vi "HFRR ADV v034 new software.vi"() -> ()   [LabVIEW 2025] (continued)
          }
        }
      }
    }
    n1885 = case shown="True" "Prog Uno" {
      frame False {
      }
      frame True {
        n1886 = stacked-sequence {
          frame #0 {
            n1887 = Delete(path (use dialog)=path "C:/LAB-IQ-NXT/UNOCOMPILE.bat" ("working directory")) -> ()  [unwired: 4 in, 3 out]
          }
          frame #1 {
            n1888 = local read "Com Port 1"() -> (w2646:refnum<visa-resource-name>)
            n1889 = Concatenate Strings("cmd.exe /c \"mode " ("command line"), w2646, ":1200,n,8,1\"\n" ("command line")) -> (w2651:string)
            n1890 = Concatenate Strings(w2651, "CD\\\nCD WinDucom\navrdude -C avrdude.conf -v -patmega328p -carduino -P" ("command line"), w2646, " -b115200 -D -Uflash:w:UNO_V20.hex:i\n" ("command line"), "\r") -> (w2653:string)
            "STR" <- w2653
            n1891 = call <vilib>:"Write Characters To File.vi"("append to file? (new file:F)"=FALSE, "character string"=w2653, "file path (dialog if empty)"=path "C:/LAB-IQ/UNOCOMPILE.bat" ("working directory")) -> ()  [unwired: 2 in, 1 out]
          }
          frame #2 {
            n1892 = disable-structure shown="Disabled" {
              frame Disabled {
                w2657 = "cmd.exe  /c \"C:\\LAB-IQ-NXT\\UNOCOMPILE.bat\"" ("string")
                n1893 = local write "Prog Uno"(FALSE ("run minimized? (F)")) -> ()
                n1894 = call <vilib>:"System Exec.vi"("expected output size  (4096)"=u32 65535, "run minimized? (F)"=FALSE, "wait until completion? (T)"=TRUE ("run minimized? (F)"), "working directory"=path "C:/LAB-IQ-NXT", "standard input"=w2657, "command line"=w2657) -> ("error out"=w2656:errorcluster, "standard output"=→"String 42":string)  [unwired: 2 in, 2 out]
                "error out 3" <- w2656
                n1895 = flat-sequence {
                  tunnel: w2656 -> [_]
                  frame #0 {
                  }
                }
              }
              frame Enabled {
              }
            }
          }
        }
      }
    }
    n1896 = case shown="\"ISO 12156\"" "TEST STANDARD" {
      frame "ASTM D6079", Default {
        w2626 = 50.0 ("Hz")
        w2627 = 53.0 ("Set Rh")
        w2629 = 1.0 ("Set Strk")
        w2628 = 60.0 ("Set Temp")
        # "astm hide"
        n1897 = local write "NORMAL LOAD"(200.0 ("NORMAL LOAD")) -> ()
        n1898 = local write "Set Strk"(w2629) -> ()
        n1899 = local write "Set Hz"(w2626) -> ()
        n1900 = local write "Set Temp"(w2628) -> ()
        n1901 = local write "Set Rh"(w2627) -> ()
        n1902 = local write "test time"(75.0 ("test time")) -> ()
        n1903 = local write "Set Stroke:"(w2629) -> ()
        n1904 = local write "Set Humidity:"(w2627) -> ()
        n1905 = local write "Set Frequency:"(w2626) -> ()
        n1906 = local write "Set Temperature:"(w2628) -> ()
        "Test Standard" <- "ASTM D6079" ("Test Standard 2")
      }
      frame "ISO 12156" {
        n1907 = local write "Set Strk"(1.0 ("Set Strk")) -> ()
        n1908 = local write "NORMAL LOAD"(200.0 ("NORMAL LOAD")) -> ()
        n1909 = local write "Set Temp"(60.0 ("Set Temp")) -> ()
        n1910 = local write "test time"(75.0 ("test time")) -> ()
        n1911 = local write "Set Hz"(50.0 ("Hz")) -> ()
        n1912 = local write "Set Rh"(53.0 ("Set Rh")) -> ()
      }
      frame "CEC F-096-A-06" {
        n1913 = local write "Set Strk"(1.0 ("Set Strk")) -> ()
        n1914 = local write "NORMAL LOAD"(200.0 ("NORMAL LOAD")) -> ()
        n1915 = local write "Set Temp"(60.0 ("Set Temp")) -> ()
        n1916 = local write "test time"(75.0 ("test time")) -> ()
        n1917 = local write "Set Hz"(50.0 ("Hz")) -> ()
        n1918 = local write "Set Rh"(53.0 ("Set Rh")) -> ()
      }
      frame "Custom" {
      }
    }
    n1919 = Or(x=w2179, y=w2177) -> (x .or. y?=w2178:bool)
    n1920 = case shown="\"About\"" w2176 {
      tunnel: [T28."Acquire" ("Main Tab") T28."Compare Files" ("Main Tab") T28."About" ("Main Tab")] -> w2187
      frame "Acquire", Default {
      }
      frame "Compare Files" {
      }
      frame "About" {
      }
    }
    n1921 = Or(x=w2182, y="OPEN") -> (x .or. y?=w2183:bool)
    n1922 = case shown="True" w2183 {
      tunnel: w2182 -> [_ w2215]
      frame False {
      }
      frame True {
        n1923 = stacked-sequence {
          tunnel: w2215 -> [_ w2282 _ _]
          frame #0 {
            w2231 = "  " ("String 6")
            n1924 = local write "OPEN"(FALSE ("open")) -> ()
            n1925 = local read "string1 2"() -> (w2219:string)
            n1926 = local read "string1 3"() -> (w2218:string)
            n1927 = local read "string1 4"() -> (w2217:string)
            n1928 = property on="OPEN" class="Bool (strict)"("Visible"=FALSE) -> ()  [unwired: 2 in, 2 out]
            n1929 = local write "String 6"(w2231) -> ()
            n1930 = local write "String 7"(w2231) -> ()
            n1931 = local write "String 8"(w2231) -> ()
            n1932 = local write "String 12"(w2231) -> ()
            n1933 = local read "OK Button 16"() -> (w2216:bool)
            n1934 = String To Path(string=w2219) -> (path=w2227:path)
            n1935 = String To Path(string=w2218) -> (path=w2226:path)
            n1936 = String To Path(string=w2217) -> (path=w2225:path)
            n1937 = case shown="True" w2216 {
              tunnel: [w2232 w2233] -> w2220
              frame False {
                n1938 = local read "string1"() -> (w2232:string)
              }
              frame True {
                n1939 = local read "String Indicator 4"() -> (w2233:string)
              }
            }
            n1940 = Open/Create/Replace File "Open File"(file path (use dialog)=w2227) -> (refnum out=w2223:refnum<file>)  [unwired: 5 in, 2 out]
            n1941 = Open/Create/Replace File "Open File"(file path (use dialog)=w2226) -> (refnum out=w2222:refnum<file>)  [unwired: 5 in, 2 out]
            n1942 = Open/Create/Replace File "Open File"(file path (use dialog)=w2225) -> (refnum out=w2221:refnum<file>)  [unwired: 5 in, 2 out]
            n1943 = while {
              tunnel: w2223 -> [w2245]
              i -> [w2241]
              stop <- w2240 continue-if-true
              (unwired) TRUE ("line mode (F)")
              n1944 = Read from Text File "Read File"(file (use dialog)=w2245) -> (text=w2242:string)  [unwired: 3 in, 3 out]
              n1945 = local write "Numeric 11"(w2241) -> ()
              n1946 = String Length(string=w2242) -> (length=w2244:i32)
              n1947 = Greater?(x=w2244, y=1) -> (0:w2240:bool)
            }
            n1948 = while {
              tunnel: w2222 -> [w2251]
              i -> [w2247]
              stop <- w2246 continue-if-true
              (unwired) TRUE ("line mode (F)")
              n1949 = Read from Text File "Read File"(file (use dialog)=w2251) -> (text=w2248:string)  [unwired: 3 in, 3 out]
              n1950 = local write "Numeric 12"(w2247) -> ()
              n1951 = String Length(string=w2248) -> (length=w2250:i32)
              n1952 = Greater?(x=w2250, y=1) -> (0:w2246:bool)
            }
            n1953 = while {
              tunnel: w2221 -> [w2257]
              i -> [w2253]
              stop <- w2252 continue-if-true
              (unwired) TRUE ("line mode (F)")
              n1954 = Read from Text File "Read File"(file (use dialog)=w2257) -> (text=w2254:string)  [unwired: 3 in, 3 out]
              n1955 = local write "Numeric 13"(w2253) -> ()
              n1956 = String Length(string=w2254) -> (length=w2256:i32)
              n1957 = Greater?(x=w2256, y=1) -> (0:w2252:bool)
            }
            n1958 = String To Path(string=w2220) -> (path=w2228:path)
            n1959 = Open/Create/Replace File "Open File"(file path (use dialog)=w2228) -> (refnum out=w2224:refnum<file>)  [unwired: 5 in, 2 out]
            n1960 = while {
              tunnel: w2224 -> [w2239]
              i -> [w2235]
              stop <- w2234 continue-if-true
              (unwired) TRUE ("line mode (F)")
              n1961 = Read from Text File "Read File"(file (use dialog)=w2239) -> (text=w2236:string)  [unwired: 3 in, 3 out]
              n1962 = local write "Numeric 8"(w2235) -> ()
              n1963 = String Length(string=w2236) -> (length=w2238:i32)
              n1964 = Greater?(x=w2238, y=1) -> (0:w2234:bool)
            }
          }
          frame #1 {
            w2409 = FALSE ("ACTUAL   MERGE")
            # "Sample Temp"
            # "ECR"
            # "COF"
            # "Time\nCOF\nFF\nTemp"
            n1965 = case shown="True" w2282 {
              tunnel: [w2429 w2430] -> w2283
              frame False {
                n1966 = local read "string1"() -> (w2429:string)
              }
              frame True {
                n1967 = local read "String Indicator 4"() -> (w2430:string)
              }
            }
            n1968 = local read "string1 3"() -> (w2327:string)
            n1969 = String To Path(string=w2283) -> (path=w2414:path)
            n1970 = String To Path(string=w2327) -> (path=w2425:path)
            n1971 = local read "Numeric 12"() -> (w2411:i32)
            n1972 = local read "Numeric 8"() -> (w2413:i32)
            n1973 = local read "string1 2"() -> (w2328:string)
            n1974 = local read "string1 4"() -> (w2326:string)
            n1975 = Open/Create/Replace File "Open File"(file path (use dialog)=w2414) -> (refnum out=w2428:refnum<file>, error out=w2427:errorcluster)  [unwired: 5 in, 1 out]
            n1976 = Open/Create/Replace File "Open File"(file path (use dialog)=w2425) -> (refnum out=w2421:refnum<file>, error out=w2422:errorcluster)  [unwired: 5 in, 1 out]
            n1977 = for {
              N: w2413 -> [_]
              tunnel: w2428 -> [w2576]
              tunnel: w2427 -> [w2575]
              tunnel: [w2565] -> w2340 mode=indexing
              tunnel: [w2563] -> w2397 mode=indexing
              tunnel: [w2564] -> w2392 mode=indexing
              tunnel: w2409 -> [_]
              tunnel: [w2557] -> w2394 mode=indexing
              tunnel: [w2553] -> w2363 mode=indexing
              tunnel: [w2549] -> w2338 mode=indexing
              tunnel: [w2545] -> w2319 mode=indexing
              tunnel: [w2540] -> w2279 mode=indexing
              (unwired) TRUE ("line mode (F)")
              # "freq"
              # "Stroke"
              # "Time"
              # "CoF"
              # "Humidity"
              # "Temp"
              # "Air Temp"
              # "ECR"
              n1978 = Read from Text File "Read File"(file (use dialog)=w2576, error in=w2575) -> (text=w2541:string)  [unwired: 2 in, 3 out]
              n1979 = local write "String 6"(w2541) -> ()
              n1980 = String Subset(string=w2541, offset (0)=0, length (rest)=14 ("length (rest)")) -> (substring=w2569:string)
              n1981 = String Subset(string=w2541, offset (0)=35, length (rest)=9 ("length (rest)")) -> (substring=w2566:string)
              n1982 = String Subset(string=w2541, offset (0)=15, length (rest)=9 ("length (rest)")) -> (substring=w2572:string)
              n1983 = Fract/Exp String To Number(string=w2569) -> (number=w2565:dbl)  [unwired: 3 in, 1 out]
              n1984 = Fract/Exp String To Number(string=w2566) -> (number=w2564:dbl)  [unwired: 3 in, 1 out]
              n1985 = Fract/Exp String To Number(string=w2572) -> (number=w2563:dbl)  [unwired: 3 in, 1 out]
              n1986 = String Subset(string=w2541, offset (0)=85, length (rest)=9 ("length (rest)")) -> (substring=w2542:string)
              n1987 = String Subset(string=w2541, offset (0)=25, length (rest)=9 ("length (rest)")) -> (substring=w2548:string)
              n1988 = String Subset(string=w2541, offset (0)=55, length (rest)=9 ("length (rest)")) -> (substring=w2550:string)
              n1989 = String Subset(string=w2541, offset (0)=45, length (rest)=9 ("length (rest)")) -> (substring=w2556:string)
              n1990 = String Subset(string=w2541, offset (0)=65, length (rest)=9 ("length (rest)")) -> (substring=w2562:string)
              n1991 = Fract/Exp String To Number(string=w2548) -> (number=w2545:dbl)  [unwired: 3 in, 1 out]
              n1992 = Fract/Exp String To Number(string=w2542) -> (number=w2540:dbl)  [unwired: 3 in, 1 out]
              n1993 = Fract/Exp String To Number(string=w2550) -> (number=w2549:dbl)  [unwired: 3 in, 1 out]
              n1994 = Fract/Exp String To Number(string=w2556) -> (number=w2553:dbl)  [unwired: 3 in, 1 out]
              n1995 = Fract/Exp String To Number(string=w2562) -> (number=w2559:dbl)  [unwired: 3 in, 1 out]
              n1996 = Add(x=w2559, y=0.0) -> (x+y=w2557:dbl)
            }
            n1997 = for {
              N: w2411 -> [_]
              tunnel: w2422 -> [w2502]
              tunnel: w2421 -> [w2501]
              tunnel: [w2491] -> w2380 mode=indexing
              tunnel: [w2489] -> w2378 mode=indexing
              tunnel: [w2490] -> w2374 mode=indexing
              tunnel: w2409 -> [_]
              tunnel: [w2483] -> w2376 mode=indexing
              tunnel: [w2479] -> w2358 mode=indexing
              tunnel: [w2475] -> w2334 mode=indexing
              tunnel: [w2472] -> w2315 mode=indexing
              tunnel: [w2468] -> w2274 mode=indexing
              (unwired) 9 ("length (rest)")
              (unwired) 9 ("length (rest)")
              (unwired) TRUE ("line mode (F)")
              n1998 = Read from Text File "Read File"(file (use dialog)=w2501, error in=w2502) -> (text=w2469:string)  [unwired: 2 in, 3 out]
              n1999 = local write "String 8"(w2469) -> ()
              n2000 = String Subset(string=w2469, offset (0)=85) -> (substring=w2471:string)  [unwired: 1 in]
              n2001 = String Subset(string=w2469, offset (0)=35, length (rest)=9 ("length (rest)")) -> (substring=w2492:string)
              n2002 = String Subset(string=w2469, offset (0)=55, length (rest)=9 ("length (rest)")) -> (substring=w2477:string)
              n2003 = String Subset(string=w2469, offset (0)=25) -> (substring=w2473:string)  [unwired: 1 in]
              n2004 = String Subset(string=w2469, offset (0)=15, length (rest)=9 ("length (rest)")) -> (substring=w2498:string)
              n2005 = String Subset(string=w2469, offset (0)=0, length (rest)=14 ("length (rest)")) -> (substring=w2495:string)
              n2006 = String Subset(string=w2469, offset (0)=45, length (rest)=9 ("length (rest)")) -> (substring=w2482:string)
              n2007 = String Subset(string=w2469, offset (0)=65, length (rest)=9 ("length (rest)")) -> (substring=w2488:string)
              n2008 = Fract/Exp String To Number(string=w2471) -> (number=w2468:dbl)  [unwired: 3 in, 1 out]
              n2009 = Fract/Exp String To Number(string=w2492) -> (number=w2490:dbl)  [unwired: 3 in, 1 out]
              n2010 = Fract/Exp String To Number(string=w2477) -> (number=w2475:dbl)  [unwired: 3 in, 1 out]
              n2011 = Fract/Exp String To Number(string=w2473) -> (number=w2472:dbl)  [unwired: 3 in, 1 out]
              n2012 = Fract/Exp String To Number(string=w2498) -> (number=w2489:dbl)  [unwired: 3 in, 1 out]
              n2013 = Fract/Exp String To Number(string=w2495) -> (number=w2491:dbl)  [unwired: 3 in, 1 out]
              n2014 = Fract/Exp String To Number(string=w2482) -> (number=w2479:dbl)  [unwired: 3 in, 1 out]
              n2015 = Fract/Exp String To Number(string=w2488) -> (number=w2485:dbl)  [unwired: 3 in, 1 out]
              n2016 = Add(x=w2485, y=0.0) -> (x+y=w2483:dbl)
            }
            n2017 = String To Path(string=w2328) -> (path=w2426:path)
            n2018 = String To Path(string=w2326) -> (path=w2420:path)
            n2019 = local read "Numeric 11"() -> (w2410:i32)
            n2020 = local read "Numeric 13"() -> (w2412:i32)
            n2021 = Open/Create/Replace File "Open File"(file path (use dialog)=w2426) -> (refnum out=w2424:refnum<file>, error out=w2423:errorcluster)  [unwired: 5 in, 1 out]
            n2022 = Open/Create/Replace File "Open File"(file path (use dialog)=w2420) -> (refnum out=w2419:refnum<file>, error out=w2418:errorcluster)  [unwired: 5 in, 1 out]
            n2023 = for {
              N: w2410 -> [_]
              tunnel: w2424 -> [w2539]
              tunnel: w2423 -> [w2538]
              tunnel: [w2528] -> w2390 mode=indexing
              tunnel: [w2526] -> w2388 mode=indexing
              tunnel: [w2527] -> w2383 mode=indexing
              tunnel: w2409 -> [_]
              tunnel: [w2520] -> w2385 mode=indexing
              tunnel: [w2516] -> w2361 mode=indexing
              tunnel: [w2512] -> w2336 mode=indexing
              tunnel: [w2508] -> w2317 mode=indexing
              tunnel: [w2503] -> w2275 mode=indexing
              (unwired) TRUE ("line mode (F)")
              n2024 = Read from Text File "Read File"(file (use dialog)=w2539, error in=w2538) -> (text=w2504:string)  [unwired: 2 in, 3 out]
              n2025 = local write "String 7"(w2504) -> ()
              n2026 = String Subset(string=w2504, offset (0)=85, length (rest)=9 ("length (rest)")) -> (substring=w2507:string)
              n2027 = String Subset(string=w2504, offset (0)=35, length (rest)=9 ("length (rest)")) -> (substring=w2529:string)
              n2028 = String Subset(string=w2504, offset (0)=55, length (rest)=9 ("length (rest)")) -> (substring=w2515:string)
              n2029 = String Subset(string=w2504, offset (0)=25, length (rest)=9 ("length (rest)")) -> (substring=w2509:string)
              n2030 = String Subset(string=w2504, offset (0)=45, length (rest)=9 ("length (rest)")) -> (substring=w2517:string)
              n2031 = String Subset(string=w2504, offset (0)=0, length (rest)=14 ("length (rest)")) -> (substring=w2532:string)
              n2032 = String Subset(string=w2504, offset (0)=15, length (rest)=9 ("length (rest)")) -> (substring=w2535:string)
              n2033 = String Subset(string=w2504, offset (0)=65, length (rest)=9 ("length (rest)")) -> (substring=w2521:string)
              n2034 = Fract/Exp String To Number(string=w2507) -> (number=w2503:dbl)  [unwired: 3 in, 1 out]
              n2035 = Fract/Exp String To Number(string=w2529) -> (number=w2527:dbl)  [unwired: 3 in, 1 out]
              n2036 = Fract/Exp String To Number(string=w2515) -> (number=w2512:dbl)  [unwired: 3 in, 1 out]
              n2037 = Fract/Exp String To Number(string=w2509) -> (number=w2508:dbl)  [unwired: 3 in, 1 out]
              n2038 = Fract/Exp String To Number(string=w2517) -> (number=w2516:dbl)  [unwired: 3 in, 1 out]
              n2039 = Fract/Exp String To Number(string=w2532) -> (number=w2528:dbl)  [unwired: 3 in, 1 out]
              n2040 = Fract/Exp String To Number(string=w2535) -> (number=w2526:dbl)  [unwired: 3 in, 1 out]
              n2041 = Fract/Exp String To Number(string=w2521) -> (number=w2524:dbl)  [unwired: 3 in, 1 out]
              n2042 = Add(x=w2524, y=0.0) -> (x+y=w2520:dbl)
            }
            n2043 = for {
              N: w2412 -> [_]
              tunnel: w2419 -> [w2467]
              tunnel: w2418 -> [w2466]
              tunnel: [w2456] -> w2372 mode=indexing
              tunnel: [w2455] -> w2365 mode=indexing
              tunnel: w2409 -> [_]
              tunnel: [w2444] -> w2370 mode=indexing
              tunnel: [w2449] -> w2367 mode=indexing
              tunnel: [w2445] -> w2357 mode=indexing
              tunnel: [w2440] -> w2332 mode=indexing
              tunnel: [w2436] -> w2313 mode=indexing
              tunnel: [w2431] -> w2273 mode=indexing
              (unwired) 1.0 ("x")
              (unwired) TRUE ("line mode (F)")
              n2044 = Read from Text File "Read File"(file (use dialog)=w2467, error in=w2466) -> (text=w2432:string)  [unwired: 2 in, 3 out]
              n2045 = local write "String 12"(w2432) -> ()
              n2046 = String Subset(string=w2432, offset (0)=85, length (rest)=9 ("length (rest)")) -> (substring=w2434:string)
              n2047 = String Subset(string=w2432, offset (0)=35, length (rest)=9 ("length (rest)")) -> (substring=w2457:string)
              n2048 = String Subset(string=w2432, offset (0)=55, length (rest)=9 ("length (rest)")) -> (substring=w2442:string)
              n2049 = String Subset(string=w2432, offset (0)=25, length (rest)=9 ("length (rest)")) -> (substring=w2438:string)
              n2050 = String Subset(string=w2432, offset (0)=45, length (rest)=9 ("length (rest)")) -> (substring=w2447:string)
              n2051 = String Subset(string=w2432, offset (0)=15, length (rest)=9 ("length (rest)")) -> (substring=w2463:string)
              n2052 = String Subset(string=w2432, offset (0)=0, length (rest)=14 ("length (rest)")) -> (substring=w2460:string)
              n2053 = String Subset(string=w2432, offset (0)=65, length (rest)=9 ("length (rest)")) -> (substring=w2450:string)
              n2054 = Fract/Exp String To Number(string=w2434) -> (number=w2431:dbl)  [unwired: 3 in, 1 out]
              n2055 = Fract/Exp String To Number(string=w2457) -> (number=w2455:dbl)  [unwired: 3 in, 1 out]
              n2056 = Fract/Exp String To Number(string=w2442) -> (number=w2440:dbl)  [unwired: 3 in, 1 out]
              n2057 = Fract/Exp String To Number(string=w2438) -> (number=w2436:dbl)  [unwired: 3 in, 1 out]
              n2058 = Fract/Exp String To Number(string=w2447) -> (number=w2445:dbl)  [unwired: 3 in, 1 out]
              n2059 = Fract/Exp String To Number(string=w2463) -> (number=w2444:dbl)  [unwired: 3 in, 1 out]
              n2060 = Fract/Exp String To Number(string=w2460) -> (number=w2456:dbl)  [unwired: 3 in, 1 out]
              n2061 = Fract/Exp String To Number(string=w2450) -> (number=w2453:dbl)  [unwired: 3 in, 1 out]
              n2062 = Add(x=w2453, y=0.0) -> (x+y=w2449:dbl)
            }
            n2063 = Delete From Array(array=w2315, index=0) -> (array with subset deleted=w2288:dbl[])  [unwired: 1 in, 1 out]
            n2064 = Delete From Array(array=w2378, index=0) -> (array with subset deleted=w2351:dbl[])  [unwired: 1 in, 1 out]
            n2065 = Delete From Array(array=w2358, index=0) -> (array with subset deleted=w2346:dbl[])  [unwired: 1 in, 1 out]
            n2066 = Delete From Array(array=w2376, index=0) -> (array with subset deleted=w2377:dbl[])  [unwired: 1 in, 1 out]
            n2067 = call-poly <vilib>:"Mean.vi"("X"=w2288) -> ("mean"=→"КОФ2 4":dbl)  [unwired: 1 out]
            n2068 = call-poly <vilib>:"Mean.vi"("X"=w2351) -> ("mean"=→"КОФ3":dbl)  [unwired: 1 out]
            n2069 = call-poly <vilib>:"Mean.vi"("X"=w2346) -> ("mean"=→"CP3":dbl)  [unwired: 1 out]
            n2070 = Delete From Array(array=w2340, index=0) -> (array with subset deleted=w2267:dbl[])  [unwired: 1 in, 1 out]
            n2071 = Delete From Array(array=w2279, index=0) -> (array with subset deleted=w2266:dbl[])  [unwired: 1 in, 1 out]
            n2072 = Delete From Array(array=w2319, index=0) -> (array with subset deleted=w2290:dbl[])  [unwired: 1 in, 1 out]
            n2073 = Delete From Array(array=w2397, index=0) -> (array with subset deleted=w2352:dbl[])  [unwired: 1 in, 1 out]
            n2074 = Delete From Array(array=w2363, index=0) -> (array with subset deleted=w2348:dbl[])  [unwired: 1 in, 1 out]
            "array w/ subset deleted" <- w2348
            n2075 = Delete From Array(array=w2394, index=0) -> (array with subset deleted=w2395:dbl[])  [unwired: 1 in, 1 out]
            n2076 = call-poly <vilib>:"Mean.vi"("X"=w2290) -> ("mean"=→"КОФ2 2":dbl)  [unwired: 1 out]
            n2077 = call-poly <vilib>:"Mean.vi"("X"=w2352) -> ("mean"=→"КОФ1":dbl)  [unwired: 1 out]
            n2078 = Bundle "Bundle"(w2267, w2266) -> (w2272:cluster{dbl[], dbl[]})  [unwired: 1 in]
            n2079 = Bundle "Bundle"(w2267, w2395) -> (w2259:cluster{dbl[], dbl[]})  [unwired: 1 in]
            n2080 = Delete From Array(array=w2274, index=0) -> (array with subset deleted=w2262:dbl[])  [unwired: 1 in, 1 out]
            n2081 = Delete From Array(array=w2275, index=0) -> (array with subset deleted=w2264:dbl[])  [unwired: 1 in, 1 out]
            n2082 = Delete From Array(array=w2385, index=0) -> (array with subset deleted=w2386:dbl[])  [unwired: 1 in, 1 out]
            n2083 = Delete From Array(array=w2273, index=0) -> (array with subset deleted=w2260:dbl[])  [unwired: 1 in, 1 out]
            n2084 = Delete From Array(array=w2367, index=0) -> (array with subset deleted=w2368:dbl[])  [unwired: 1 in, 1 out]
            n2085 = Delete From Array(array=w2392, index=0) -> (array with subset deleted=w2298:dbl[])  [unwired: 1 in, 1 out]
            n2086 = Delete From Array(array=w2338, index=0) -> (array with subset deleted=w2294:dbl[])  [unwired: 1 in, 1 out]
            n2087 = Delete From Array(array=w2374, index=0) -> (array with subset deleted=w2296:dbl[])  [unwired: 1 in, 1 out]
            n2088 = Delete From Array(array=w2334, index=0) -> (array with subset deleted=w2292:dbl[])  [unwired: 1 in, 1 out]
            n2089 = Delete From Array(array=w2383, index=0) -> (array with subset deleted=w2297:dbl[])  [unwired: 1 in, 1 out]
            n2090 = Delete From Array(array=w2336, index=0) -> (array with subset deleted=w2293:dbl[])  [unwired: 1 in, 1 out]
            n2091 = Delete From Array(array=w2317, index=0) -> (array with subset deleted=w2289:dbl[])  [unwired: 1 in, 1 out]
            n2092 = Delete From Array(array=w2361, index=0) -> (array with subset deleted=w2347:dbl[])  [unwired: 1 in, 1 out]
            n2093 = Delete From Array(array=w2388, index=0) -> (array with subset deleted=w2349:dbl[])  [unwired: 1 in, 1 out]
            n2094 = Delete From Array(array=w2365, index=0) -> (array with subset deleted=w2295:dbl[])  [unwired: 1 in, 1 out]
            n2095 = Delete From Array(array=w2332, index=0) -> (array with subset deleted=w2291:dbl[])  [unwired: 1 in, 1 out]
            n2096 = Delete From Array(array=w2313, index=0) -> (array with subset deleted=w2287:dbl[])  [unwired: 1 in, 1 out]
            n2097 = Delete From Array(array=w2357, index=0) -> (array with subset deleted=w2345:dbl[])  [unwired: 1 in, 1 out]
            n2098 = Delete From Array(array=w2370, index=0) -> (array with subset deleted=w2350:dbl[])  [unwired: 1 in, 1 out]
            n2099 = Delete From Array(array=w2380, index=0) -> (array with subset deleted=w2263:dbl[])  [unwired: 1 in, 1 out]
            n2100 = Delete From Array(array=w2390, index=0) -> (array with subset deleted=w2265:dbl[])  [unwired: 1 in, 1 out]
            n2101 = Delete From Array(array=w2372, index=0) -> (array with subset deleted=w2261:dbl[])  [unwired: 1 in, 1 out]
            n2102 = Bundle "Bundle"(w2267, w2298) -> (w2285:cluster{dbl[], dbl[]})  [unwired: 1 in]
            n2103 = Bundle "Bundle"(w2267, w2352) -> (w2286:cluster{dbl[], dbl[]})  [unwired: 1 in]
            n2104 = Bundle "Bundle"(w2298, w2294) -> (w2300:cluster{dbl[], dbl[]})  [unwired: 1 in]
            n2105 = Bundle "Bundle"(w2263, w2262) -> (w2270:cluster{dbl[], dbl[]})  [unwired: 1 in]
            n2106 = Bundle "Bundle"(w2296, w2292) -> (w2302:cluster{dbl[], dbl[]})  [unwired: 1 in]
            n2107 = Bundle "Bundle"(w2263, w2296) -> (w2406:cluster{dbl[], dbl[]})  [unwired: 1 in]
            n2108 = Bundle "Bundle"(w2263, w2292) -> (w2330:cluster{dbl[], dbl[]})  [unwired: 1 in]
            n2109 = Bundle "Bundle"(w2263, w2351) -> (w2416:cluster{dbl[], dbl[]})  [unwired: 1 in]
            n2110 = Bundle "Bundle"(w2263, w2346) -> (w2354:cluster{dbl[], dbl[]})  [unwired: 1 in]
            n2111 = Bundle "Bundle"(w2263, w2377) -> (w2401:cluster{dbl[], dbl[]})  [unwired: 1 in]
            n2112 = Bundle "Bundle"(w2297, w2293) -> (w2301:cluster{dbl[], dbl[]})  [unwired: 1 in]
            n2113 = Bundle "Bundle"(w2265, w2264) -> (w2271:cluster{dbl[], dbl[]})  [unwired: 1 in]
            n2114 = Bundle "Bundle"(w2265, w2297) -> (w2408:cluster{dbl[], dbl[]})  [unwired: 1 in]
            n2115 = Bundle "Bundle"(w2265, w2293) -> (w2331:cluster{dbl[], dbl[]})  [unwired: 1 in]
            n2116 = Bundle "Bundle"(w2265, w2347) -> (w2355:cluster{dbl[], dbl[]})  [unwired: 1 in]
            n2117 = Bundle "Bundle"(w2265, w2349) -> (w2417:cluster{dbl[], dbl[]})  [unwired: 1 in]
            n2118 = Bundle "Bundle"(w2265, w2386) -> (w2399:cluster{dbl[], dbl[]})  [unwired: 1 in]
            n2119 = Bundle "Bundle"(w2295, w2291) -> (w2303:cluster{dbl[], dbl[]})  [unwired: 1 in]
            n2120 = Bundle "Bundle"(w2261, w2260) -> (w2269:cluster{dbl[], dbl[]})  [unwired: 1 in]
            n2121 = Bundle "Bundle"(w2261, w2295) -> (w2407:cluster{dbl[], dbl[]})  [unwired: 1 in]
            n2122 = Bundle "Bundle"(w2261, w2291) -> (w2329:cluster{dbl[], dbl[]})  [unwired: 1 in]
            n2123 = Bundle "Bundle"(w2261, w2345) -> (w2353:cluster{dbl[], dbl[]})  [unwired: 1 in]
            n2124 = Bundle "Bundle"(w2261, w2350) -> (w2415:cluster{dbl[], dbl[]})  [unwired: 1 in]
            n2125 = Bundle "Bundle"(w2261, w2368) -> (w2400:cluster{dbl[], dbl[]})  [unwired: 1 in]
            n2126 = call-poly <vilib>:"Mean.vi"("X"=w2348) -> ("mean"=→"CP1":dbl)  [unwired: 1 out]
            n2127 = call-poly <vilib>:"Mean.vi"("X"=w2289) -> ("mean"=→"КОФ2 3":dbl)  [unwired: 1 out]
            n2128 = call-poly <vilib>:"Mean.vi"("X"=w2347) -> ("mean"=→"CP2":dbl)  [unwired: 1 out]
            n2129 = call-poly <vilib>:"Mean.vi"("X"=w2349) -> ("mean"=→"КОФ2":dbl)  [unwired: 1 out]
            n2130 = call-poly <vilib>:"Mean.vi"("X"=w2287) -> ("mean"=→"КОФ2 5":dbl)  [unwired: 1 out]
            n2131 = call-poly <vilib>:"Mean.vi"("X"=w2345) -> ("mean"=→"CP4":dbl)  [unwired: 1 out]
            n2132 = call-poly <vilib>:"Mean.vi"("X"=w2350) -> ("mean"=→"КОФ4":dbl)  [unwired: 1 out]
            n2133 = Bundle "Bundle"(w2267, w2294) -> (w2258:cluster{dbl[], dbl[]})  [unwired: 1 in]
            n2134 = Bundle "Bundle"(w2267, w2348) -> (w2281:cluster{dbl[], dbl[]})  [unwired: 1 in]
            n2135 = Build Array "Build Array"(w2258, w2281) -> (w2284:cluster{dbl[], dbl[]}[])
            "XY Graph 17" <- w2284
            n2136 = Build Array "Build Array"(w2272, w2271, w2270, w2269) -> (→"Frequency ( Hz )":cluster{dbl[], dbl[]}[])
            n2137 = Build Array "Build Array"(w2300, w2301, w2302, w2303) -> (→"Air Temp ( °C ) vs Humidity ( % RH )":cluster{dbl[], dbl[]}[])
            n2138 = Build Array "Build Array"(w2285, w2408, w2406, w2407) -> (→"Air Temperature  ( °C )":cluster{dbl[], dbl[]}[])
            n2139 = Build Array "Build Array"(w2258, w2331, w2330, w2329) -> (→"Humidity ( %RH )":cluster{dbl[], dbl[]}[])
            n2140 = Build Array "Build Array"(w2286, w2417, w2416, w2415) -> (→"Coefficient Of Friction":cluster{dbl[], dbl[]}[])
            n2141 = Build Array "Build Array"(w2281, w2355, w2354, w2353) -> (→"Sample Temperature ( °C )":cluster{dbl[], dbl[]}[])
            n2142 = Build Array "Build Array"(w2259, w2399, w2401, w2400) -> (→"XY Graph 13":cluster{dbl[], dbl[]}[])
            n2143 = Bundle "Bundle"(w2267, w2290) -> (w2312:cluster{dbl[], dbl[]})  [unwired: 1 in]
            n2144 = Bundle "Bundle"(w2263, w2288) -> (w2310:cluster{dbl[], dbl[]})  [unwired: 1 in]
            n2145 = Bundle "Bundle"(w2265, w2289) -> (w2311:cluster{dbl[], dbl[]})  [unwired: 1 in]
            n2146 = Bundle "Bundle"(w2261, w2287) -> (w2309:cluster{dbl[], dbl[]})  [unwired: 1 in]
            n2147 = Build Array "Build Array"(w2312, w2311, w2310, w2309) -> (→"Stroke ( mm )":cluster{dbl[], dbl[]}[])
            n2148 = local write "XY Graph 16"(w2284) -> ()
          }
          frame #2 {
          }
          frame #3 {
            n2149 = local write "Numeric 8"(0 ("Numeric 8")) -> ()
            n2150 = local write "Numeric 11"(0 ("Numeric 11")) -> ()
            n2151 = local write "Numeric 12"(0 ("Numeric 12")) -> ()
            n2152 = local write "Numeric 13"(0 ("Numeric 13")) -> ()
            n2153 = property on="OPEN" class="Bool (strict)"("Visible"=TRUE) -> ()  [unwired: 2 in, 2 out]
            n2154 = local read "String Control 2"() -> (w2584:string)
            n2155 = local read "String Control 4"() -> (w2583:string)
            n2156 = local read "String Control 6"() -> (w2582:string)
            n2157 = local read "String Control 8"() -> (w2581:string)
            n2158 = Match Pattern(string=w2584, regular expression="Samples / cycle :- ") -> (after substring=w2598:string)  [unwired: 1 in, 3 out]
            n2159 = Match Pattern(string=w2584, regular expression="Frequency :- ") -> (after substring=w2617:string)  [unwired: 1 in, 3 out]
            n2160 = Match Pattern(string=w2583, regular expression="Samples / cycle :- ") -> (after substring=w2594:string)  [unwired: 1 in, 3 out]
            n2161 = Match Pattern(string=w2583, regular expression="Frequency :- ") -> (after substring=w2612:string)  [unwired: 1 in, 3 out]
            n2162 = Match Pattern(string=w2582, regular expression="Samples / cycle :- ") -> (after substring=w2590:string)  [unwired: 1 in, 3 out]
            n2163 = Match Pattern(string=w2582, regular expression="Frequency :- ") -> (after substring=w2607:string)  [unwired: 1 in, 3 out]
            n2164 = Match Pattern(string=w2581, regular expression="Samples / cycle :- ") -> (after substring=w2586:string)  [unwired: 1 in, 3 out]
            n2165 = Match Pattern(string=w2581, regular expression="Frequency :- ") -> (after substring=w2602:string)  [unwired: 1 in, 3 out]
            n2166 = String Subset(string=w2598, length (rest)=6 ("length (rest)")) -> (substring=w2600:string)  [unwired: 1 in]
            n2167 = String Subset(string=w2617, length (rest)=9 ("length (rest)")) -> (substring=w2619:string)  [unwired: 1 in]
            n2168 = String Subset(string=w2594, length (rest)=6 ("length (rest)")) -> (substring=w2596:string)  [unwired: 1 in]
            n2169 = String Subset(string=w2612, length (rest)=9 ("length (rest)")) -> (substring=w2614:string)  [unwired: 1 in]
            n2170 = String Subset(string=w2590, length (rest)=6 ("length (rest)")) -> (substring=w2592:string)  [unwired: 1 in]
            n2171 = String Subset(string=w2607, length (rest)=9 ("length (rest)")) -> (substring=w2609:string)  [unwired: 1 in]
            n2172 = String Subset(string=w2586, length (rest)=6 ("length (rest)")) -> (substring=w2588:string)  [unwired: 1 in]
            n2173 = String Subset(string=w2602, length (rest)=9 ("length (rest)")) -> (substring=w2604:string)  [unwired: 1 in]
            n2174 = Fract/Exp String To Number(string=w2600) -> (number=w2580:dbl)  [unwired: 3 in, 1 out]
            n2175 = Fract/Exp String To Number(string=w2619) -> (number=w2620:dbl)  [unwired: 3 in, 1 out]
            n2176 = Fract/Exp String To Number(string=w2596) -> (number=w2579:dbl)  [unwired: 3 in, 1 out]
            n2177 = Fract/Exp String To Number(string=w2614) -> (number=w2615:dbl)  [unwired: 3 in, 1 out]
            n2178 = Fract/Exp String To Number(string=w2592) -> (number=w2578:dbl)  [unwired: 3 in, 1 out]
            n2179 = Fract/Exp String To Number(string=w2609) -> (number=w2610:dbl)  [unwired: 3 in, 1 out]
            n2180 = Fract/Exp String To Number(string=w2588) -> (number=w2577:dbl)  [unwired: 3 in, 1 out]
            n2181 = Fract/Exp String To Number(string=w2604) -> (number=w2605:dbl)  [unwired: 3 in, 1 out]
            n2182 = local write "sample1"(w2580) -> ()
            n2183 = local write "freq1"(w2620) -> ()
            n2184 = local write "sample2"(w2579) -> ()
            n2185 = local write "freq2"(w2615) -> ()
            n2186 = local write "sample3"(w2578) -> ()
            n2187 = local write "freq3"(w2610) -> ()
            n2188 = local write "sample4"(w2577) -> ()
            n2189 = local write "freq 4"(w2605) -> ()
          }
        }
      }
    }
    n2190 = case shown="True" w2178 {
      selector: w2178 -> [_ w2197]
      frame False {
      }
      frame True {
        n2191 = Not(x=w2197) -> (.not. x?=w2193:bool)
        n2192 = local write "service 3"(w2193) -> ()
        n2193 = local write "OPEN 6"(w2193) -> ()
        n2194 = call <vilib>:"System Exec.vi"("wait until completion? (T)"=TRUE, "command line"="C:\\LAB-IQ\\Scar View.exe") -> ("error out"=→"error out 5":errorcluster)  [unwired: 6 in, 3 out]
      }
    }
    n2195 = case shown="\"Acquire\", Default" w2187 {
      frame "Acquire", Default {
        # "Elapsed time\ncof\nstroke\nAir temp\nTemp\nHumidity"
        n2196 = disable-structure shown="Disabled" {
          frame Disabled {
            n2197 = local read "Flag"() -> (w2896:dbl)
            n2198 = local read "RUN"() -> (w2893:bool)
            n2199 = Not(x=w2893) -> (.not. x?=w2892:bool)
            n2200 = Equal?(x=w2896, y=10.0) -> (x = y?=w2894:bool)
            n2201 = And(x=w2894, y=w2892) -> (x .and. y?=w2891:bool)
            n2202 = case shown="True" w2891 {
              frame False {
              }
              frame True {
                w2897 = FALSE ("Heater Button")
                n2203 = local write "Humidity"(w2897) -> ()
                n2204 = local write "Heater Button"(w2897) -> ()
              }
            }
          }
          frame Enabled {
          }
        }
        n2205 = disable-structure shown="Disabled" {
          frame Disabled {
            n2206 = case shown="True" {
              selector: _ -> [_ _]
              frame False {
              }
              frame True {
                w2950 = TRUE ("Heater")
                n2207 = local write "Humidity"(w2950) -> ()
                n2208 = local write "Heater Button"(w2950) -> ()
                n2209 = local read "TEST STANDARD"() -> (w2953:T3)
                n2210 = local read "TEST STANDARD"() -> (w2948:T3)
                n2211 = Equal?(x=w2953, y=enum16{"ASTM D6079", "ISO 12156", "Custom"}."ISO 12156" ("Test Standard")) -> (x = y?=w2951:bool)
                n2212 = Equal?(x=w2948, y=enum16{"ASTM D6079", "ISO 12156", "Custom"}."ASTM D6079" ("Test Standard")) -> (x = y?=w2947:bool)
                n2213 = case shown="True" w2951 {
                  frame False {
                  }
                  frame True {
                    n2214 = local write "airtempflg"(FALSE ("airtempflg")) -> ()
                    n2215 = local write item#-1(TRUE ("Heater")) -> ()
                  }
                }
                n2216 = case shown="True" w2947 {
                  frame False {
                  }
                  frame True {
                    n2217 = local write "airtempflg"(TRUE ("airtempflg")) -> ()
                    n2218 = local write item#-1(FALSE ("Heater")) -> ()
                  }
                }
              }
            }
          }
          frame Enabled {
          }
        }
        n2219 = stacked-sequence {
          frame #0 {
            n2220 = case shown="True" "RST FF" {
              frame False {
              }
              frame True {
                w2967 = 0.0 ("X Scale.Range:Maximum")
                n2221 = property on="Frictional Force ( N )" class="WFChart (strict)"("XScale.Maximum"=600.0 ("X Scale.Range:Maximum"), "XScale.Minimum"=w2967, "YScale.Maximum"=10.0 ("Y Scale.Range:Maximum"), "YScale.Minimum"=w2967) -> ()  [unwired: 2 in, 2 out]
              }
            }
          }
          frame #1 {
            n2222 = case shown="True" "RST TEMP" {
              frame False {
              }
              frame True {
                n2223 = property on="Temperature ( Deg C )" class="WFChart (strict)"("XScale.Minimum"=0.0 ("X Scale.Range:Minimum"), "XScale.Maximum"=600.0 ("X Scale.Range:Maximum"), "YScale.Minimum"=0.0 ("Y Scale.Range:Minimum"), "YScale.Maximum"=100.0 ("Y Scale.Range:Maximum")) -> ()  [unwired: 2 in, 2 out]
              }
            }
          }
          frame #2 {
            n2224 = case shown="True" "RSTCOF" {
              frame False {
              }
              frame True {
                n2225 = property on="Coefficient of Friction" class="WFChart (strict)"("XScale.Minimum"=0.0 ("X Scale.Range:Minimum"), "XScale.Maximum"=600.0 ("X Scale.Range:Maximum"), "YScale.Maximum"=1.0 ("X Scale.Range:Minimum"), "YScale.Minimum"=0.0 ("X Scale.Range:Minimum")) -> ()  [unwired: 2 in, 2 out]
              }
            }
          }
          frame #3 {
            n2226 = case shown="True" "RSTCOF 2" {
              frame False {
              }
              frame True {
                (unwired) 100.0 ("Y Scale.Range:Maximum")
                (unwired) 0.0 ("Y Scale.Range:Minimum")
                (unwired) 600.0 ("X Scale.Range:Maximum")
                (unwired) 0.0 ("X Scale.Range:Minimum")
              }
            }
          }
          frame #4 {
            n2227 = case shown="True" "RSTCOF 3" {
              frame False {
              }
              frame True {
                n2228 = property on="Electrical Contact Resistance ( % )" class="WFChart (strict)"("XScale.Minimum"=0.0 ("X Scale.Range:Minimum"), "XScale.Maximum"=600.0 ("X Scale.Range:Maximum"), "YScale.Minimum"=0.0 ("Y Scale.Range:Minimum"), "YScale.Maximum"=100.0 ("Y Scale.Range:Maximum")) -> ()  [unwired: 2 in, 2 out]
              }
            }
          }
        }
        n2229 = local read "RUN"() -> (w2886:bool)
        n2230 = case shown="False" w2886 {
          frame False {
          }
          frame True {
          }
        }
        n2231 = local read "RUN"() -> (w2890:bool)
        n2232 = case shown="False" w2890 {
          tunnel: [FALSE ("TEST RUNNING") TRUE ("TEST RUNNING")] -> w2889
          frame False {
            w2986 = 0.0 ("Flag")
            n2233 = local write "Elapsed time"(0.0 ("elapsedtime")) -> ()
            n2234 = local write "Time Remaining"(w2986) -> ()
            n2235 = local write "Flag"(w2986) -> ()
            n2236 = local write "Remaining Time"(w2986) -> ()
          }
          frame True {
            n2237 = local write "Flag"(10.0 ("Flag")) -> ()
          }
        }
        n2238 = local read "AIR TEMP"() -> (w2884:dbl)
        n2239 = Greater Or Equal?(x=w2884, y=15.0) -> (x >= y?=w2885:bool)
        "powstat" <- w2885
        n2240 = case shown="True" "Save & Continue" {
          frame False {
          }
          frame True {
            n2241 = local read "USER ID"() -> (w3288:string)
            n2242 = local read "FILE"() -> (w3296:string)
            n2243 = String Length(string=w3296) -> (length=w3294:i32)
            n2244 = String Length(string=w3288) -> (length=w3291:i32)
            n2245 = Greater?(x=w3294, y=0) -> (0:w3293:bool)
            n2246 = Greater?(x=w3291, y=0) -> (0:w3290:bool)
            n2247 = And(x=w3293, y=w3290) -> (x .and. y?=w3289:bool)
            n2248 = case shown="True" w3289 {
              frame False {
                n2249 = stacked-sequence {
                  frame #0 {
                    n2250 = One Button Dialog(message="Please Enter a File Name and Operator ID to save data !", button name ("OK")="Ok") -> ()  [unwired: 1 out]
                  }
                  frame #1 {
                    n2251 = local write "Save & Continue"(FALSE ("OK Button")) -> ()
                  }
                }
                n2252 = local write "Save & Continue"(FALSE ("OK Button")) -> ()
              }
              frame True {
                n2253 = stacked-sequence {
                  frame #0 {
                    n2254 = local read "FILE"() -> (w3302:string)
                    n2255 = call "file check.vi"("file name in"=w3302) -> ("file name out"=w3301:string)  [unwired: 9 in, 1 out]
                    n2256 = call <vilib>:"Application Directory.vi"() -> ("Application Directory"=w3312:path)
                    n2257 = Build Path(base path=w3312, name or relative path="data") -> (appended path=w3311:path)
                    n2258 = call <vilib>:"Trim Whitespace.vi"("string"=w3301) -> ("trimmed string"=w3309:string)  [unwired: 1 in]
                    n2259 = call <vilib>:"Trim Whitespace.vi"("string"=w3301) -> ("trimmed string"=w3310:string)  [unwired: 1 in]
                    n2260 = List Folder(path=w3311) -> (folder names=w3307:string[])  [unwired: 3 in, 3 out]
                    n2261 = Match Pattern(string=w3309, regular expression="_(") -> (before substring=w3306:string)  [unwired: 1 in, 3 out]
                    n2262 = for {
                      tunnel: w3307 -> [w3321] mode=indexing
                      tunnel: w3306 -> [w3319]
                      shift-right: [w3317] -> w3304
                      shift-left: bool[] [] -> [w3318]
                      n2263 = Match Pattern(string=w3321, regular expression="_(") -> (before substring=w3320:string)  [unwired: 1 in, 3 out]
                      n2264 = Equal?(x=w3320, y=w3319) -> (x = y?=w3316:bool)
                      n2265 = case shown="True" w3316 {
                        tunnel: w3316 -> [_ w3324]
                        tunnel: w3318 -> [w3323 w3326]
                        tunnel: [w3323 w3325] -> w3317
                        frame False {
                        }
                        frame True {
                          n2266 = Insert Into Array(array=w3326, new element=w3324) -> (w3325:bool[])  [unwired: 1 in]
                        }
                      }
                    }
                    n2267 = Equal?(x=w3307, y=w3306) -> (x = y?=w3315:bool[])
                    n2268 = Or Array Elements(Boolean array=w3315) -> (logical OR=w3314:bool)
                    n2269 = Array Size(array=w3304) -> (size(s)=w3303:i32)
                    n2270 = case shown="True" w3314 {
                      tunnel: w3310 -> [_ w3334]
                      tunnel: w3303 -> [_ w3327]
                      frame False {
                      }
                      frame True {
                        n2271 = Number To Decimal String(number=w3327) -> (decimal integer string=w3330:string)  [unwired: 1 in]
                        n2272 = Search/Split String(string=w3334, search string/char (-)="_(" ("regular expression")) -> (substring before match=w3332:string)  [unwired: 1 in, 2 out]
                        n2273 = Concatenate Strings(w3332, "_(" ("regular expression"), w3330, ")" ("regular expression")) -> (w3328:string)
                        n2274 = local write "FILE"(w3328) -> ()
                      }
                    }
                  }
                  frame #1 {
                    w3337 = 0.0
                    w3350 = cluster{"y":dbl, dbl, "y":dbl}[] [] ("History Data")
                    w3351 = FALSE ("Heater Button")
                    (unwired) ")!" ("string")
                    (unwired) ")" ("string")
                    w3349 = dbl[] [] ("History Data")
                    w3355 = "\r"
                    # "C:\\WinDucom\\Data\\"
                    # "C:\\LAB-IQ-NXT\\data"
                    n2275 = local write "Humidity ( %RH )"(w3337) -> ()
                    n2276 = local write "Frequency ( Hz )"(w3337) -> ()
                    n2277 = local write "Stroke 3"(w3337) -> ()
                    n2278 = local write "speedop"(0.0 ("PIDclk 2")) -> ()
                    n2279 = local write "Set Temp 2"(65.0 ("Set Temp 2")) -> ()
                    n2280 = local write "AIR TEMP"(w3337) -> ()
                    n2281 = local write "clk"(0.0 ("clk")) -> ()
                    n2282 = local write "Stroke 4"(w3337) -> ()
                    n2283 = local write "COF 2"(w3337) -> ()
                    n2284 = local write "TEMP"(w3337) -> ()
                    n2285 = local write "ecr 3"(w3337) -> ()
                    n2286 = local write "FF 3"(w3337) -> ()
                    n2287 = local write "FF 2"(w3337) -> ()
                    n2288 = property on="Humidity ( %RH )" class="WFChart (strict)"("History Data"=w3349) -> ()  [unwired: 2 in, 2 out]
                    n2289 = property on="Coefficient of Friction" class="WFChart (strict)"("History Data"=w3349) -> ()  [unwired: 2 in, 2 out]
                    n2290 = property on="Coefficient of Friction" class="WFChart (strict)"("History Data"=w3349) -> ()  [unwired: 2 in, 2 out]
                    n2291 = property on="Frictional Force ( N )" class="WFChart (strict)"("History Data"=w3349) -> ()  [unwired: 2 in, 2 out]
                    n2292 = property on="Electrical Contact Resistance ( % )" class="WFChart (strict)"("History Data"=w3349) -> ()  [unwired: 2 in, 2 out]
                    n2293 = property on="Electrical Contact Resistance ( % )" class="WFChart (strict)"("History Data"=w3349) -> ()  [unwired: 2 in, 2 out]
                    n2294 = property on="Temperature ( Deg C )" class="WFChart (strict)"("History Data"=w3349) -> ()  [unwired: 2 in, 2 out]
                    n2295 = property on="Frictional Force ( N )" class="WFChart (strict)"("History Data"=w3349) -> ()  [unwired: 2 in, 2 out]
                    n2296 = property on="Coefficient of Friction" class="WFChart (strict)"("History Data"=w3349) -> ()  [unwired: 2 in, 2 out]
                    n2297 = property on="Frictional Force ( N )" class="WFChart (strict)"("History Data"=w3349) -> ()  [unwired: 2 in, 2 out]
                    n2298 = property on="Electrical Contact Resistance ( % )" class="WFChart (strict)"("History Data"=w3349) -> ()  [unwired: 2 in, 2 out]
                    n2299 = property on="Temperature ( Deg C )" class="WFChart (strict)"("History Data"=w3349) -> ()  [unwired: 2 in, 2 out]
                    n2300 = property on="Humidity ( %RH )" class="WFChart (strict)"("History Data"=w3349) -> ()  [unwired: 2 in, 2 out]
                    n2301 = property on="Stroke ( mm )" class="WFChart (strict)"("History Data"=w3350) -> ()  [unwired: 2 in, 2 out]
                    n2302 = property on="Stroke ( mm )" class="WFChart (strict)"("History Data"=w3350) -> ()  [unwired: 2 in, 2 out]
                    n2303 = local write "Humidity"(w3351) -> ()
                    n2304 = local write "Heater Button"(w3351) -> ()
                    n2305 = local read "FILE"() -> (w3345:string)
                    n2306 = disable-structure shown="Enabled" {
                      disable-tunnel: [w3389 _] -> w3336
                      frame Enabled {
                        n2307 = local read "NORMAL LOAD"() -> (w3389:dbl)
                      }
                      frame Disabled {
                      }
                    }
                    n2308 = call "file check.vi"("file name in"=w3345) -> ("error out"=w3348:errorcluster, "file name out"=w3342:string)  [unwired: 9 in]
                    n2309 = call "FILE PATH CREATION.vi"("error in"=w3348, "FILE NAME :"=w3342) -> ("FILE OUT"=w3341:path)  [unwired: 8 in, 1 out]
                    n2310 = Concatenate Strings(w3342, ".dgf" ("Substring")) -> (w3347:string)
                    n2311 = Concatenate Strings(w3342, ".duf" ("Substring")) -> (w3343:string)
                    n2312 = Multiply(x=w3336, y=1.0) -> (x*y=w3368:dbl)
                    n2313 = Build Path(base path=w3341, name or relative path=w3347) -> (appended path=w3340:path)
                    n2314 = Build Path(base path=w3341, name or relative path=w3343) -> (appended path=w3339:path)
                    n2315 = Number To Fractional String(number=w3368, width (-)=i16 5, precision (6)=i16 2) -> (F-format string=w3376:string)  [unwired: 1 in]
                    n2316 = local read "tested by"() -> (w3335:string)
                    n2317 = local read "Fuel Discription :"() -> (w3364:string)
                    n2318 = local read "Batch Ref Num :"() -> (w3353:string)
                    n2319 = Get Date/Time String(date format (0)=enum16{"short", "long", "abbreviated"}."short") -> (date string=w3387:string, time string=w3384:string)  [unwired: 2 in]
                    n2320 = local read "Remarks :"() -> (w3363:string)
                    n2321 = Concatenate Strings("Load :- " ("Substring"), w3376, " grams ," ("Substring")) -> (w3375:string)
                    n2322 = local read "String 41"() -> (w3356:string)
                    n2323 = Concatenate Strings(w3364) -> (w3365:string)
                    n2324 = Concatenate Strings(w3353) -> (w3352:string)
                    n2325 = Concatenate Strings(w3335) -> (w3359:string)
                    n2326 = Concatenate Strings("(" ("Substring"), w3387, ")" ("Substring"), w3384) -> (w3358:string)
                    "concatenated string" <- w3358
                    n2327 = Concatenate Strings(w3363, "," ("string")) -> (w3362:string)
                    n2328 = Concatenate Strings("  TIME;      COF;       STROKE;     AIR TEMP;  TEMP;  HUMIDITY;  ECR; PID-OUT; FREQUENCY" ("Substring"), "\r") -> (w3371:string)
                    n2329 = Concatenate Strings(w3356, w3355, "Fuel Discription :-" ("Substring"), w3365, w3355, w3375, w3355, "Batch Ref Num :-" ("Substring"), w3352, w3355, " Remarks :- " ("Substring"), w3362, w3355, " Date :- " ("Substring"), w3358, w3355, "Tested By :-" ("Substring"), w3359) -> (w3369:string)
                    "REMARKS" <- w3369
                    n2330 = call <vilib>:"Write Characters To File.vi"("append to file? (new file:F)"=FALSE, "character string"=w3371, "file path (dialog if empty)"=w3340) -> ()  [unwired: 2 in, 1 out]
                    n2331 = call <vilib>:"Write Characters To File.vi"("append to file? (new file:F)"=FALSE, "character string"=w3369, "file path (dialog if empty)"=w3339) -> ()  [unwired: 2 in, 1 out]
                  }
                  frame #2 {
                    n2332 = local write "Cycles elapsed"(0 ("Cycles elapsed")) -> ()
                    n2333 = local write "cyclecount"(0 ("cyclecount")) -> ()
                    n2334 = local write "Save & Continue"(FALSE ("OK")) -> ()
                    n2335 = local write "autostrtflg"(TRUE ("autostrtflg")) -> ()
                    n2336 = local write "Save"(FALSE ("Save")) -> ()
                    n2337 = Get Date/Time In Seconds() -> (seconds since 1Jan1904=w3394:timestamp)
                    n2338 = To Double Precision Float(number=w3394) -> (double precision float=w3393:dbl)
                    n2339 = local write "acq timer"(w3393) -> ()
                    n2340 = One Button Dialog(message="Please ensure sample is mounted properly and machine is ready in all aspects for testing !", button name ("OK")="Ok") -> ()  [unwired: 1 out]
                  }
                  frame #3 {
                    n2341 = stacked-sequence {
                      frame #0 {
                        n2342 = local write "Main Dashboard Buttons"(T1."Dashboard" ("Main Dashboard Buttons")) -> ()
                        n2343 = local write "Main Tab"(T2."Acquire" ("Main Tab")) -> ()
                      }
                      frame #1 {
                        n2344 = local write "EVENT LOG"("" ("EVENT LOG")) -> ()
                      }
                      frame #2 {
                        n2345 = Wait (ms)(milliseconds to wait=u32 50) -> ()  [unwired: 1 out]
                      }
                      frame #3 {
                        n2346 = disable-structure shown="Disabled" {
                          frame Disabled {
                            n2347 = local read "EVENT LOG"() -> (w3406:string)
                            n2348 = call "Event Log.vi"("Content"="Test Details", "EVENT LOG"=w3406) -> ("EVENT LOG"=w3405:string)  [unwired: 8 in, 1 out]
                            n2349 = local write "EVENT LOG"(w3405) -> ()
                          }
                          frame Enabled {
                          }
                        }
                      }
                      frame #4 {
                        n2350 = Wait (ms)(milliseconds to wait=u32 50) -> ()  [unwired: 1 out]
                      }
                      frame #5 {
                        n2351 = local read "FILE"() -> (w3408:string)
                        n2352 = Concatenate Strings("File Name :" ("Content"), w3408) -> (w3409:string)
                        n2353 = local read "EVENT LOG"() -> (w3412:string)
                        n2354 = call "Event Log.vi"("Content"=w3409, "EVENT LOG"=w3412) -> ("EVENT LOG"=w3411:string)  [unwired: 8 in, 1 out]
                        n2355 = local write "EVENT LOG"(w3411) -> ()
                      }
                      frame #6 {
                        n2356 = Wait (ms)(milliseconds to wait=u32 50) -> ()  [unwired: 1 out]
                      }
                      frame #7 {
                        n2357 = local read "Batch Ref Num :"() -> (w3414:string)
                        n2358 = Concatenate Strings("Batch Ref No :" ("Content"), w3414) -> (w3415:string)
                        n2359 = local read "EVENT LOG"() -> (w3418:string)
                        n2360 = call "Event Log.vi"("Content"=w3415, "EVENT LOG"=w3418) -> ("EVENT LOG"=w3417:string)  [unwired: 8 in, 1 out]
                        n2361 = local write "EVENT LOG"(w3417) -> ()
                      }
                      frame #8 {
                        n2362 = Wait (ms)(milliseconds to wait=u32 50) -> ()  [unwired: 1 out]
                      }
                      frame #9 {
                        n2363 = local read "tested by"() -> (w3420:string)
                        n2364 = Concatenate Strings("Tested By :" ("Content"), w3420) -> (w3421:string)
                        n2365 = local read "EVENT LOG"() -> (w3424:string)
                        n2366 = call "Event Log.vi"("Content"=w3421, "EVENT LOG"=w3424) -> ("EVENT LOG"=w3423:string)  [unwired: 8 in, 1 out]
                        n2367 = local write "EVENT LOG"(w3423) -> ()
                      }
                      frame #10 {
                        n2368 = Wait (ms)(milliseconds to wait=u32 50) -> ()  [unwired: 1 out]
                      }
                      frame #11 {
                        n2369 = local read "TEST STANDARD"() -> (w3427:T3)
                        n2370 = case shown="\"ASTM D6079\", Default" w3427 {
                          tunnel: ["ASTM D6079" "ISO 12156" "CEC F-096-A-06" "Custom"] -> w3426
                          frame "ASTM D6079", Default {
                          }
                          frame "ISO 12156" {
                          }
                          frame "CEC F-096-A-06" {
                          }
                          frame "Custom" {
                          }
                        }
                        n2371 = Concatenate Strings("Test Standard :" ("Content"), w3426) -> (w3428:string)
                        n2372 = local read "EVENT LOG"() -> (w3431:string)
                        n2373 = call "Event Log.vi"("Content"=w3428, "EVENT LOG"=w3431) -> ("EVENT LOG"=w3430:string)  [unwired: 8 in, 1 out]
                        n2374 = local write "EVENT LOG"(w3430) -> ()
                      }
                      frame #12 {
                        n2375 = Wait (ms)(milliseconds to wait=u32 50) -> ()  [unwired: 1 out]
                      }
                      frame #13 {
                        n2376 = local read "Fuel Discription :"() -> (w3437:string)
                        n2377 = Concatenate Strings("Fuel Description :" ("Content"), w3437) -> (w3438:string)
                        n2378 = local read "EVENT LOG"() -> (w3441:string)
                        n2379 = call "Event Log.vi"("Content"=w3438, "EVENT LOG"=w3441) -> ("EVENT LOG"=w3440:string)  [unwired: 8 in, 1 out]
                        n2380 = local write "EVENT LOG"(w3440) -> ()
                      }
                      frame #14 {
                        n2381 = Wait (ms)(milliseconds to wait=u32 50) -> ()  [unwired: 1 out]
                      }
                      frame #15 {
                        n2382 = local read "Remarks :"() -> (w3443:string)
                        n2383 = Concatenate Strings("Remarks :" ("Content"), w3443) -> (w3444:string)
                        n2384 = local read "EVENT LOG"() -> (w3447:string)
                        n2385 = call "Event Log.vi"("Content"=w3444, "EVENT LOG"=w3447) -> ("EVENT LOG"=w3446:string)  [unwired: 8 in, 1 out]
                        n2386 = local write "EVENT LOG"(w3446) -> ()
                      }
                      frame #16 {
                        n2387 = Wait (ms)(milliseconds to wait=u32 50) -> ()  [unwired: 1 out]
                      }
                      frame #17 {
                        n2388 = local read "USER ID"() -> (w3449:string)
                        n2389 = Concatenate Strings("Operator ID :" ("Content"), w3449) -> (w3451:string)
                        n2390 = local read "EVENT LOG"() -> (w3453:string)
                        n2391 = call "Event Log.vi"("Content"=w3451, "EVENT LOG"=w3453) -> ("EVENT LOG"=w3452:string)  [unwired: 8 in, 1 out]
                        n2392 = local write "EVENT LOG"(w3452) -> ()
                      }
                      frame #18 {
                        n2393 = Wait (ms)(milliseconds to wait=u32 50) -> ()  [unwired: 1 out]
                      }
                      frame #19 {
                        n2394 = disable-structure shown="Disabled" {
                          frame Disabled {
                            n2395 = local read "EVENT LOG"() -> (w3457:string)
                            n2396 = call "Event Log.vi"("Content"="Test Parameter", "EVENT LOG"=w3457) -> ("EVENT LOG"=w3456:string)  [unwired: 8 in, 1 out]
                            n2397 = local write "EVENT LOG"(w3456) -> ()
                          }
                          frame Enabled {
                          }
                        }
                      }
                      frame #20 {
                        n2398 = Wait (ms)(milliseconds to wait=u32 50) -> ()  [unwired: 1 out]
                      }
                      frame #21 {
                        n2399 = local read "Set Hz"() -> (w3461:dbl)
                        n2400 = Number To Fractional String(number=w3461, precision (6)=i16 2) -> (F-format string=w3460:string)  [unwired: 2 in]
                        n2401 = Concatenate Strings("Set Frequency [Hz] :" ("Content"), w3460) -> (w3463:string)
                        n2402 = local read "EVENT LOG"() -> (w3465:string)
                        n2403 = call "Event Log.vi"("Content"=w3463, "EVENT LOG"=w3465) -> ("EVENT LOG"=w3464:string)  [unwired: 8 in, 1 out]
                        n2404 = local write "EVENT LOG"(w3464) -> ()
